vi "L05.vi"() -> ()   [LabVIEW 2012]
panel:
  out "Numeric":i32
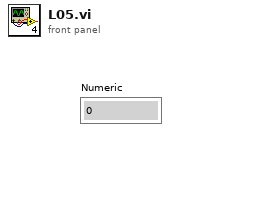
[diagram p1: front panel]
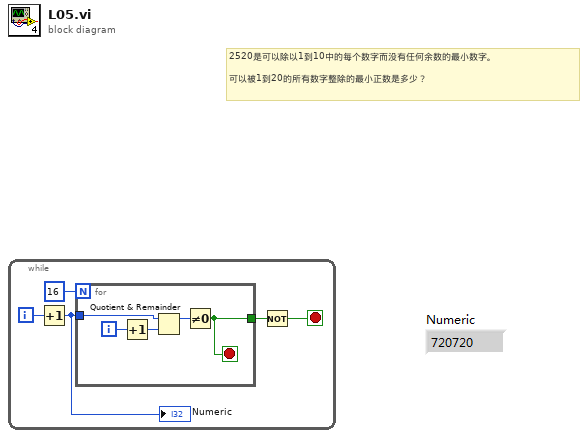
[diagram p0: block diagram]
diagram:
  # "2520是可以除以1到10中的每个数字而没有任何余数的最小数字。\n\n可以被1到20的所有数字整除的最小正数是多少？"
  n1 = while {
    i -> [w4]
    stop <- w1 stop-if-true
    n2 = Increment(x=w4) -> (x+1=w3:i32)
    "Numeric" <- w3
    n3 = for {
      N: 16 -> [_]
      tunnel: w3 -> [w10]
      tunnel: [w6] -> w2
      i -> [w9]
      stop <- w6 stop-if-true
      n4 = Increment(x=w9) -> (x+1=w8:i32)
      n5 = Quotient & Remainder(x=w10, y=w8) -> (x-y*floor(x/y)=w7:i32)  [unwired: 1 out]
      n6 = Not Equal To 0?(x=w7) -> (x != 0?=w6:bool)
    }
    n7 = Not(x=w2) -> (.not. x?=w1:bool)
  }
